vi "Dashboard Main.vi"() -> ()   [LabVIEW 2014]
uses:
  <vilib>/event_ctls.llb/eventvkey.ctl
  <vilib>/Utility/config.llb/NI_LVConfig.lvlib
  <vilib>/Utility/config.llb/Write Key (I32).vi
  <vilib>/Rock Robotics/WPI/Dashboard/WPI_DashboardLogging Global.vi
  <vilib>/Utility/config.llb/Write Key (String).vi
panel:
  in  "TCP":refnum<k5>
  out "Camera IP":string
  out "Image Message":string="Timeout in Camera Communications"
  in  "Dashboard Tab":T1(tab)
  out "RightPwr":dbl(slide) scale=-100.0..100.0
  out "RightSpd":dbl(slide) scale=-12.0..12.0
  out "LeftSpd":dbl(slide) scale=-12.0..12.0
  out "LeftPwr":dbl(slide) scale=-100.0..100.0
  in  "Camera Settings":T2={"Frame Rate"=30, "Compression"=30, "Size"=1} {"Frame Rate" scale=1.0..30.0; "Size" items=["640x480", "320x240", "160x120"]}
  out "MotorChart R":cluster{"Numeric":dbl, "Numeric":dbl}(graph)
  out "MotorChart L":T3(graph)
  out "MotorSliders R":cluster{"MotorSlide1":dbl, "MotorSlide2":dbl} {"MotorSlide2" scale=-1.0..1.0 scale format="%#_2e"; "MotorSlide1" scale=-1.0..1.0 scale format="%#_2e"}
  out "MotorSliders L":T4 {"MotorSlide4 2" scale=0.0..14.0 scale format="%#_2e"; "MotorSlide2" scale=-1.0..1.0 scale format="%#_2e"; "MotorSlide1" scale=-1.0..1.0 scale format="%#_2e"}
  out "JS1 Z":dbl(slide) scale=-1.0..1.0 scale format="%#_2e"
  out "JS1 Graph":cluster{"X":dbl, "Y":dbl}[](graph)
  out "JS1 Buttons":T5
  out "JS2 Z":dbl(slide) scale=-1.0..1.0 scale format="%#_2e"
  out "JS2 Graph":cluster{"X":dbl, "Y":dbl}[](graph)
  out "JS2 Buttons":T5
  out "Mode":T6(ring)=enum."Auto Disabled"
  in  "DB Camera Config":bool
  out "fps":dbl format="%#.1g"
  out "Mbps":dbl format="%#.1g"
  out "Mbps 2":bool
  in  "DB/String 9":string
  in  "DB/String 8":string
  in  "DB/String 7":string
  in  "DB/String 6":string
  in  "DB/String 5":string
  in  "DB/String 4":string
  in  "DB/String 3":string
  in  "DB/String 2":string
  in  "DB/String 1":string
  in  "DB/String 0":string
  in  "DB/Slider 0":dbl(slide) scale=0.0..5.0
  in  "DB/Slider 1":dbl(slide) scale=0.0..5.0
  in  "DB/Slider 2":dbl(slide) scale=0.0..5.0
  in  "DB/Slider 3":dbl(slide) scale=0.0..5.0
  out "DB/LED 3":bool
  out "DB/LED 2":bool
  out "DB/LED 1":bool
  out "DB/LED 0":bool
  in  "DB/Button 3":bool
  in  "DB/Button 2":bool
  in  "DB/Button 1":bool
  in  "DB/Button 0":bool caption="New Name"
  in  "Test Slider":dbl(slide) scale=0.0..100.0 scale format="%#_3g"
  in  "On/Off":bool caption="Solenoid"
  in  "Test Name":u16(ring) items=["Select the test to run...", "Example Test", "-------------------------------", "List of tests is built in robot code.", "Replace with your own automated tests."]
  in  "Test Tree":string(tree)
  in  "Motor":cluster{"Value":dbl, "Enable":bool} {"Value" scale=-1.0..1.0 scale format="%#_3g"}
  out "Progress":T7 {"Test Progress" scale=0.0..100.0}
  in  "Rev/Fwd":cluster{"Forward":bool, "Reverse":bool}
  in  "Test Ring":u16(ring) items=["Monochrome", "Color"]
  in  "Listbox":i32(listbox)
  out "Tree":string(tree)
  out "Boolean":bool
  # "Left"
  # "Front"
  # "Right"
  # "Battery"
  # "This tab is a great place for autonomous settings and robot-specific values.\nPlace controls and indicators inside this tab and match name to\nDashboard Variables on robot. You can also delete this comment."
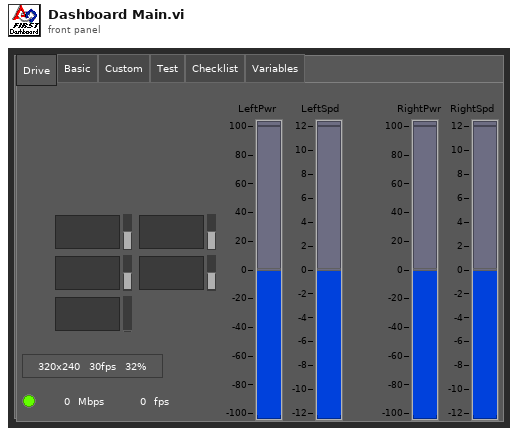
[diagram p1: front panel]
types:
  T1 = enum32{"Drive", "Basic", "Custom", "Test", "Checklist", "Variables"}
  T2 = cluster{"Frame Rate":i32, "Compression":i32, "Size":u16}
  T3 = cluster{"Numeric":dbl, "Numeric":dbl, "Battery V":dbl}
  T4 = cluster{"MotorSlide1":dbl, "MotorSlide2":dbl, "MotorSlide4 2":dbl}
  T5 = cluster{bool, bool, bool, bool, bool, bool, bool, bool, bool, bool, bool, bool}
  T6 = enum8{"Tele-Op Disabled", "Tele-Op Enabled", "Auto Disabled", "Auto Enabled", "Test Disabled", "Test Enabled", "Disconnected", "No Code", "E-Stop"}
  T7 = cluster{"Test Progress":u8, "Test Progress Text":string}
  T8 = typedef "Image Type" = u32
  T9 = typedef "IMAQ Image.ctl" = refnum<image>
  T10 = cluster{"Error Strings":string, "Disable Counts":cluster{u16, u16}, "Rail Faults":cluster{u16, u16, u16}, "Robot IP":string, "DB Mode":u8, "Event Info":cluster{"Name":string, "Type":u8, "Number":u16, "Replay":u8}, "Camera Addr":string}
  T11 = cluster{"Storage":cluster{"Disk Free":u64, "RAM Block":u32, "RAM free":u32}, "CPU Utilization":cluster{"CPU % ISR":sgl, "CPU % Time Crit":sgl, "CPU % Timed Str":sgl, "CPU % High":sgl, "CPU % Above":sgl, "CPU % Normal":sgl, "CPU % Low":sgl}, "CAN":cluster{"% Bus Utilization":sgl, "Bus Off Cnt":u32, "TX_FIFO Full Cnt":u32, "Receive Error Cnt":u8, "Transmit Error Cnt":u8}, "HID":cluster{"HID Outputs":u32, "Rumble Low":u16, "Rumble High":u16}[]}
  T12 = cluster{"Status bits":cluster{"Test Mode":bool, "Autonomous":bool, "Enabled":bool, "Code Start":bool, "Brownout":bool, "Reserved 2":bool, "Reserved 3":bool, "E-Stop":bool}, "Code Trace":cluster{"Disabled":bool, "TeleOp":bool, "Auto":bool, "Test":bool}, "Controller Type":enum16{"unknown", "cRIO", "roboRio"}, "Code?":enum16{"unknown", "noCode", "code"}, "Battery V":dbl}
  T13 = cluster{"Control Bits":cluster{"TestMode":bool, "Autonomous":bool, "Enabled":bool, "FMS Present":bool, bool, bool, bool, "E-Stop":bool}, "Team Station ":u8, "Countdown":sgl, "Joystick Values":cluster{"Axes":dbl[], "Buttons":bool[], "POVs":i16[]}[]}
  T14 = cluster{"Axes":dbl[], "Buttons":bool[], "POVs":i16[]}[]
  T15 = cluster{"Axes":dbl[], "Buttons":bool[], "POVs":i16[]}
  T16 = cluster{"Buttons[0]":bool, "Buttons[1]":bool, "Buttons[2]":bool, "Buttons[3]":bool, "Buttons[4]":bool, "Buttons[5]":bool, "Buttons[6]":bool, "Buttons[7]":bool, "Buttons[8]":bool, "Buttons[9]":bool, "Buttons[10]":bool, "Buttons[11]":bool}
  T17 = typedef "NI_LVConfig.lvlib/Config Data RefNum.ctl" = refnum<k1>
  T18 = cluster{"Operation":enum16{"Update", "Clear"}, "Color Box":u32}[]
  T19 = typedef "eventvkey.ctl" = enum16{"ASCII", "Enter", "Return", "Shift", "Ctrl", "Alt", "Cmd", "Opt", "Caps", "NumLock", "Clear", "Break", "Up", "Down", "Left", "Right", "Insert", "Delete", "Home", "End", "PageUp", "PageDown", "Escape", "Help", "Pause", "ScrollLock", "F1", "F2", "F3", "F4", "F5", "F6", "F7", "F8", "F9", "F10", "F11", "F12", "F13", "F14", "F15", "F16", "F17", "F18", "F19", "F20", "F21", "F22", "F23", "F24", "Play", "VolumeUp", "VolumeDown", "Mute", "Two Byte Char"}
  T20 = cluster{"Image Size":bool, "Image Type":bool, "Pixel Value":bool, "ROI Information":bool, "Zoom Factor":bool}
  T21 = enum8{"Enabled", "Disabled", "Disabled and Grayed Out"}
  T22 = cluster{"Operation":enum16{"Update", "Clear"}, "Color Box":u32}
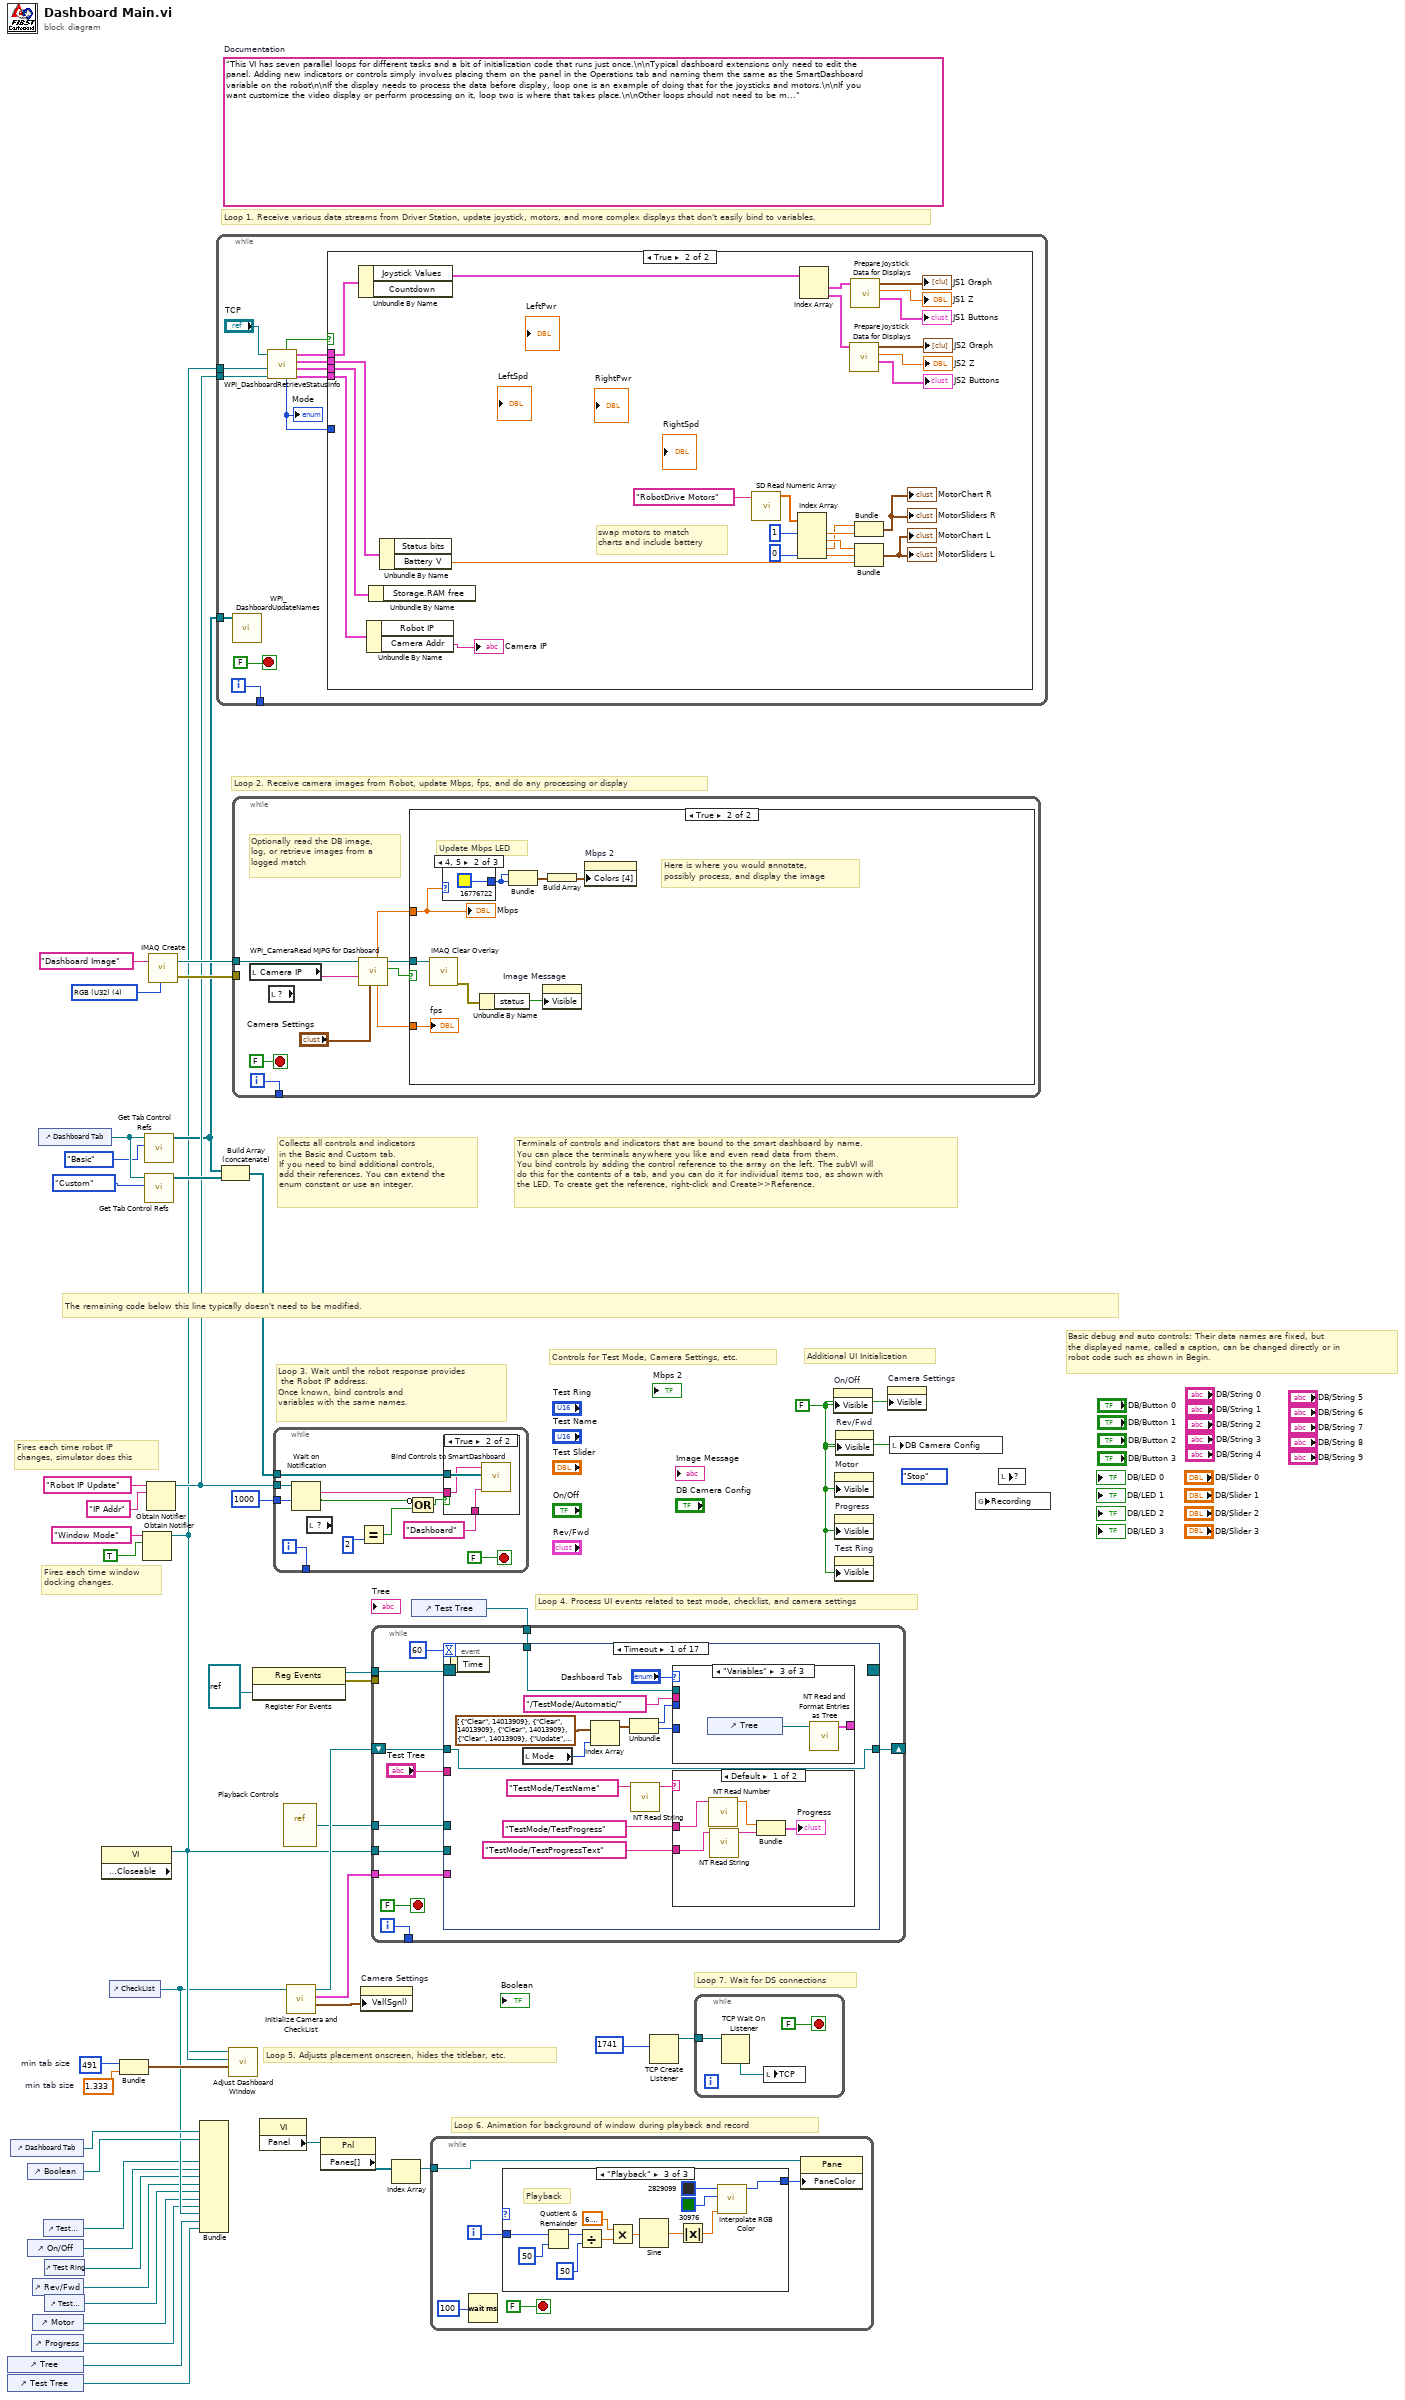
[diagram p0: block diagram]
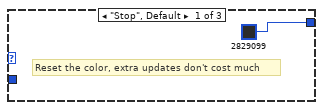
[diagram p3: hidden frame]
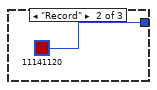
[diagram p4: hidden frame]
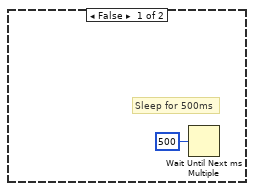
[diagram p6: hidden frame]
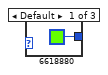
[diagram p7: hidden frame]
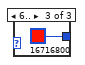
[diagram p8: hidden frame]
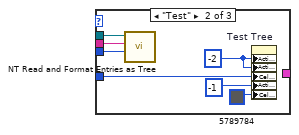
[diagram p10: hidden frame]
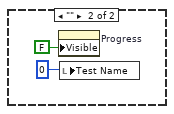
[diagram p11: hidden frame]
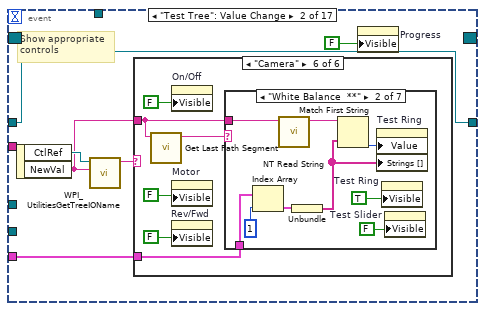
[diagram p12: hidden frame]
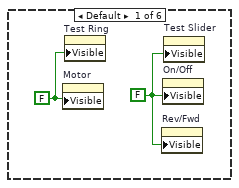
[diagram p13: hidden frame]
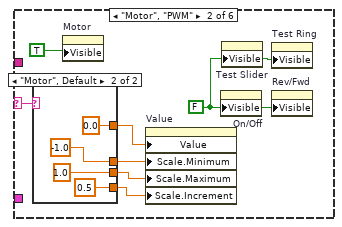
[diagram p14: hidden frame]
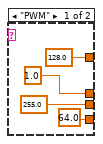
[diagram p15: hidden frame]
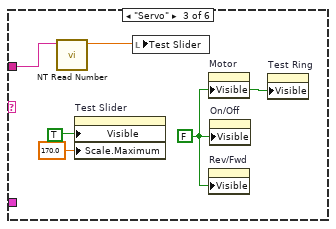
[diagram p16: hidden frame]
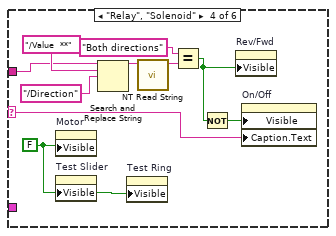
[diagram p17: hidden frame]
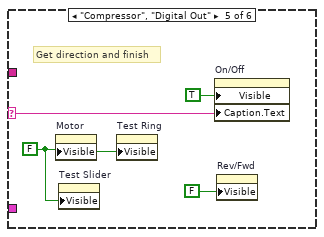
[diagram p18: hidden frame]
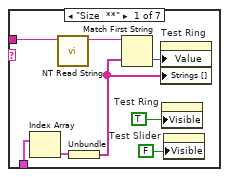
[diagram p19: hidden frame]
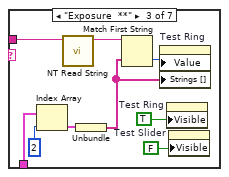
[diagram p20: hidden frame]
diagram:
  w22 = 491  # min tab size
  w21 = 1.333  # min tab size
  (unwired) enum32{"Stop", "Record", "Playback"}."Stop" ("Rec Mode")
  w6 = FALSE ("Visible")
  (unwired) "This VI has seven parallel loops for different tasks and a bit of initialization code that runs just once.\n\nTypical dashboard extensions only need to edit the panel. Adding new indicators or controls simply involves placing them on the panel in the Operations tab and naming them the same as the SmartDashboard variable on the robot\n\nIf the display needs to process the data before display, loop one is an example of doing that for the joysticks and motors.\n\nIf you want customize the video display or perform processing on it, loop two is where that takes place.\n\nOther loops should not need to be modified. They are pretty standard, and document the task they perform."  # Documentation
  w47 = T8 4 items=["Grayscale (U8)", "Grayscale (I16)", "Grayscale (SGL)", "Complex (CSG)", "RGB (U32)", "HSL (U32)", "RGB (U64)"] ("Image Type")
  # "Loop 7. Wait for DS connections"
  # "Basic debug and auto controls: Their data names are fixed, but\nthe displayed name, called a caption, can be changed directly or in\nrobot code such as shown in Begin."
  # "Controls for Test Mode, Camera Settings, etc."
  # "Additional UI Initialization"
  # "Loop 6. Animation for background of window during playback and record"
  # "Fires each time robot IP\nchanges, simulator does this"
  # "Fires each time window\ndocking changes."
  # "Collects all controls and indicators\nin the Basic and Custom tab.\nIf you need to bind additional controls,\nadd their references. You can extend the\nenum constant or use an integer."
  # "The remaining code below this line typically doesn't need to be modified."
  # "Loop 4. Process UI events related to test mode, checklist, and camera settings"
  # "Terminals of controls and indicators that are bound to the smart dashboard by name.\nYou can place the terminals anywhere you like and even read data from them.\nYou bind controls by adding the control reference to the array on the left. The subVI will\ndo this for the contents of a tab, and you can do it for individual items too, as shown with\nthe LED. To create get the reference, right-click and Create>>Reference."
  # "Loop 3. Wait until the robot response provides\n the Robot IP address.\nOnce known, bind controls and\nvariables with the same names."
  # "Loop 5. Adjusts placement onscreen, hides the titlebar, etc."
  # "Loop 1. Receive various data streams from Driver Station, update joystick, motors, and more complex displays that don't easily bind to variables."
  # "Loop 2. Receive camera images from Robot, update Mbps, fps, and do any processing or display"
  n1 = control-ref of="Tree"() -> (w15:refnum<vi>)
  n2 = control-ref of="Test Tree"() -> (w14:refnum<vi>)
  n3 = control-ref of="Dashboard Tab"() -> (w23:refnum<vi>)
  n4 = control-ref of="Boolean"() -> (w19:refnum<vi>)
  n5 = control-ref of="On/Off"() -> (w10:refnum<vi>)
  n6 = control-ref of="Progress"() -> (w7:refnum<vi>)
  n7 = control-ref of="Rev/Fwd"() -> (w8:refnum<vi>)
  n8 = control-ref of="Motor"() -> (w12:refnum<vi>)
  n9 = control-ref of="Dashboard Tab"() -> (w26:refnum<vi>)
  n10 = control-ref of="Test Slider"() -> (w11:refnum<vi>)
  n11 = control-ref of="Test Ring"() -> (w9:refnum<vi>)
  n12 = control-ref of="Test Name"() -> (w13:refnum<vi>)
  n13 = property class="VI" props=["Front Panel.Closeable"]() -> (reference out=w27:refnum<vi>)  [unwired: 2 in, 2 out]
  n14 = control-ref of="CheckList"() -> (w16:refnum<vi>)
  n15 = Bundle("min tab size"=w22, "min tab size"=w21) -> (w20:cluster{"min tab size":i32, "min tab size":dbl})  [unwired: 1 in]
  n16 = Obtain Notifier(name (unnamed)="Window Mode", notification data type=TRUE) -> (notifier out=w3:refnum<notifier>)  [unwired: 2 in, 2 out]
  n17 = call <vilib>:"Get Tab Control Refs.vi"("Page Index"=T1."Basic" ("Dashboard Tab"), "TabControl in"=w26) -> ("ControlsOnPage"=w4:refnum<vi>[])  [unwired: 9 in]
  n18 = call <vilib>:"Get Tab Control Refs.vi"("Page Index"=T1."Custom" ("Dashboard Tab"), "TabControl in"=w26) -> ("ControlsOnPage"=w25:refnum<vi>[])  [unwired: 9 in]
  n19 = Obtain Notifier(name (unnamed)="Robot IP Update", notification data type="IP Addr" ("name (unnamed)")) -> (notifier out=w5:refnum<notifier>)  [unwired: 2 in, 2 out]
  n20 = call "IMAQ Create"("Image Name"="Dashboard Image", "Image Type"=w47) -> ("New Image"=w45:T9, "error out"=w44:errorcluster)  [unwired: 2 in, 1 out]
  n21 = Bundle("Dashboard Tab"=w23, "Boolean"=w19, "Test Slider"=w11, "On/Off"=w10, "Test Ring"=w9, "Rev/Fwd"=w8, "Test Name"=w13, "Motor"=w12, "Progress"=w7, "CheckList"=w16, "Tree"=w15, "Test Tree"=w14) -> ()  [unwired: 4 in, 1 out]
  n22 = while {
    tunnel: [w58] -> _
    tunnel: w5 -> [w52]
    tunnel: w4 -> [w51]
    tunnel: w3 -> [w48]
    i -> [w58]
    stop <- FALSE stop-if-true
    n23 = call <vilib>:"WPI_DashboardUpdateNames.vi"("Controls on Tab"=w51) -> ()  [unwired: 11 in]
    n24 = call <vilib>:"WPI_DashboardRetrieveStatusInfo.vi"("Binding Refnum"=w52, "Window Mode Notifier"=w48, "TCP Cnx"="TCP") -> ("Power and Errors"=w53:T10, "Robot Metrics"=w56:T11, "Status Info"=w57:T12, "Control Info"=w54:T13, "Robot Mode"=w50:T6, "Process?"=w55:bool)  [unwired: 3 in]
    "Mode" <- w50
    n25 = case shown="True" w55 {
      tunnel: w57 -> [_ w84]
      tunnel: w56 -> [_ w83]
      tunnel: w54 -> [_ w82]
      tunnel: w53 -> [_ w81]
      tunnel: w50 -> [_ _]
      frame False {
      }
      frame True {
        # "swap motors to match\ncharts and include battery"
        n26 = Unbundle By Name(w82) -> ("Joystick Values"=w69:T14)  [unwired: 1 out]
        n27 = Unbundle By Name(w81) -> ("Camera Addr"=→"Camera IP":string)  [unwired: 1 out]
        n28 = Unbundle By Name(w83) -> ()  [unwired: 1 out]
        n29 = Unbundle By Name(w84) -> ("Battery V"=w70:dbl)  [unwired: 1 out]
        n30 = call <vilib>:"SD Read Numeric Array.vi"("Name"="RobotDrive Motors") -> ("Numeric Array"=w72:dbl[])  [unwired: 8 in, 2 out]
        n31 = Index Array(array=w72, index #1=1, index #4=0) -> (element #1=w76:dbl, element #2=w77:dbl, element #3=w75:dbl, element #4=w80:dbl)  [unwired: 2 in]
        n32 = Index Array(array=w69) -> (element #1=w68:T15, element #2=w63:T15)  [unwired: 2 in]
        n33 = call "Prepare Joystick Data for Displays.vi"("Joystick Values"=w63) -> ("Buttons"=→"JS2 Buttons":T16, "Z Axis"=→"JS2 Z":dbl, "Cartesian Data"=→"JS2 Graph":cluster{"X axis":dbl, "X axis":dbl}[])  [unwired: 8 in]
        n34 = call "Prepare Joystick Data for Displays.vi"("Joystick Values"=w68) -> ("Buttons"=→"JS1 Buttons":T16, "Z Axis"=→"JS1 Z":dbl, "Cartesian Data"=→"JS1 Graph":cluster{"X axis":dbl, "X axis":dbl}[])  [unwired: 8 in]
        n35 = Bundle("Numeric"=w75, "Numeric"=w76) -> (→"MotorChart R" →"MotorSliders R":cluster{"Numeric":dbl, "Numeric":dbl})  [unwired: 1 in]
        n36 = Bundle("Numeric"=w77, "Numeric"=w80, "Battery V"=w70) -> (→"MotorChart L" →"MotorSliders L":T3)  [unwired: 1 in]
      }
    }
  }
  n37 = Build Array (concatenate)(w4, w25) -> (w24:refnum<vi>[])
  n38 = call "Adjust Dashboard Window.vi"("Size Constraints"=w20, "VI"=w27, "Notifier in"=w3) -> ()  [unwired: 9 in]
  n39 = while {
    tunnel: w45 -> [w91]
    tunnel: w44 -> [_]
    tunnel: [w92] -> _
    i -> [w92]
    stop <- FALSE stop-if-true
    # "Optionally read the DB image,\nlog, or retrieve images from a\nlogged match"
    n40 = local read "Camera IP"() -> (w85:string)
    n41 = local read item#-1() -> ()  [unwired: 1 out]
    n42 = call <vilib>:"WPI_CameraRead MJPG for Dashboard.vi"("Camera Settings"="Camera Settings", "Camera IP"=w85, "Refnum in"=w91) -> ("Active"=w89:bool, "Refnum out"=w90:T9, "FPS"=w88:dbl, "Bandwidth (Mbps)"=w87:dbl)  [unwired: 5 in]
    n43 = case shown="True" w89 {
      tunnel: w90 -> [_ w97]
      tunnel: w87 -> [_ w96]
      tunnel: w88 -> [_ w95]
      frame False {
        # "Sleep for 500ms"
        n44 = Wait Until Next ms Multiple(millisecond multiple=u32 500) -> ()  [unwired: 1 out]
      }
      frame True {
        # "Here is where you would annotate,\npossibly process, and display the image"
        # "Update Mbps LED"
        n45 = call "IMAQ Clear Overlay"("Image"=w97) -> ("error out"=w101:errorcluster)  [unwired: 2 in, 8 out]
        n46 = case shown="4, 5" w96 {
          tunnel: [u32 6618880 ("Color Box") u32 16776722 ("Color Box") u32 16716800 ("Color Box")] -> w98
          frame Default {
          }
          frame 4, 5 {
          }
          frame 6.. {
          }
        }
        n47 = Unbundle By Name(w101) -> ("status"=w102:bool)
        n48 = Bundle("Color Box"=w98, "Color Box"=w98) -> (w100:cluster{"Color Box":u32, "Color Box":u32})  [unwired: 1 out]
        n49 = property on="Image Message" class="Str"("Visible"=w102) -> ()  [unwired: 2 in, 2 out]
        n50 = Build Array(w100) -> (w99:cluster{"Color Box":u32, "Color Box":u32}[])
        n51 = property on="Mbps 2" class="Bool (strict)"("Colors [4]"=w99) -> ()  [unwired: 2 in, 2 out]
        "Mbps" <- w96
        "fps" <- w95
      }
    }
  }
  n52 = register-events(refnum<vi> refnum) -> (reference out=w31:refnum<event-registration>, error out=w30:errorcluster)  [unwired: 2 in]
  n53 = property class="VI"() -> ("Panel"=w34:refnum<vi>)  [unwired: 2 in, 2 out]
  n54 = while {
    tunnel: w24 -> [w116]
    tunnel: w5 -> [w114]
    tunnel: [w112] -> _
    tunnel: u32 1000 ("milliseconds to wait") -> [w111]
    i -> [w112]
    stop <- FALSE stop-if-true
    n55 = Wait on Notification(notifier=w114, timeout in ms (-1)=w111) -> (notification=w113:string, timed out?=w109:bool)  [unwired: 2 in, 2 out]
    n56 = local read item#-1() -> ()  [unwired: 1 out]
    n57 = Equal?(y=u16 2 ("Rec Mode")) -> (x = y?=w108:bool)  [unwired: 1 in]
    n58 = Compound Arithmetic op=OR(invert w109, w108) -> (w110:bool)
    n59 = case shown="True" w110 {
      tunnel: w116 -> [_ w119]
      tunnel: w113 -> [_ w118]
      tunnel: "Dashboard" -> [_ w117]
      frame False {
      }
      frame True {
        n60 = call <vilib>:"Bind Controls to SmartDashboard.vi"("Client Name"=w117, "Bound Control Refs"=w119, "Server IP Address"=w118) -> ()  [unwired: 9 in]
      }
    }
  }
  n61 = vi-ref "Playback Controls.vi"() -> (w32:refnum<vi>)
  n62 = call "Initialize Camera and CheckList.vi"("ListBox in"=w16) -> ("Cluster"=w38:cluster{"value":i32, "value":i32, "index":i32}, "Array"=w39:cluster{string[]}[], "File Refnum"=w37:T17)  [unwired: 8 in]
  n63 = property class="Pnl"(reference=w34) -> ("Panes[]"=w35:refnum<vi>[])  [unwired: 1 in, 2 out]
  n64 = property on="Camera Settings" class="Clust (strict)"("Val(Sgnl)"=w38) -> ()  [unwired: 2 in, 2 out]
  n65 = Index Array(array=w35) -> (element=w33:refnum<vi>)  [unwired: 1 in]
  n66 = control-ref of="Test Tree"() -> (w36:refnum<vi>)
  n67 = while {
    tunnel: w39 -> [w127]
    shift-right: [w126] -> _
    shift-left: w37 -> [w125]
    tunnel: [w124] -> _
    tunnel: w36 -> [w123]
    tunnel: w32 -> [w122]
    tunnel: w31 -> [w121]
    tunnel: w30 -> [_]
    tunnel: w27 -> [w120]
    i -> [w124]
    stop <- FALSE stop-if-true
    n68 = event shown="[0] Timeout" {
      selector: w121 -> [_ _ _ _ _ _ _ _ _ _ _ _ _ _ _ _ _]
      dyn-events: [_ _ _ _ _ _ _ _ _ _ _ _ _ w363 _ _ _] -> _
      timeout: u32 60 ("milliseconds to wait") -> [_ _ _ _ _ _ _ _ _ _ _ _ _ _ _ _ _]
      tunnel: w123 -> [w139 _ _ _ _ _ _ _ _ _ _ _ _ _ _ _ _]
      tunnel: "Test Tree" -> [_ _ _ _ _ _ _ _ w334 w342 w344 w348 w356 _ _ _ _]
      tunnel: w127 -> [_ w161 _ _ _ _ w298 w328 _ _ _ _ _ _ _ _ _]
      tunnel: [w135 w160 w259 w264 w272 w284 w297 w321 w333 w340 w343 w347 w355 w365 w377 w378 w387] -> w126
      tunnel: w125 -> [w135 w160 w259 w264 w272 w284 w296 w321 w333 w340 w343 w347 w355 w365 w377 w378 w387]
      tunnel: w122 -> [_ _ _ _ _ _ _ _ _ _ _ _ _ w366 _ w381 _]
      tunnel: w120 -> [_ _ _ _ _ _ _ _ _ _ _ _ _ w361 _ _ _]
      event Timeout {
        n69 = event-data() -> ()  [unwired: 1 in, 1 out]
        n70 = local read "Mode"() -> (w138:T6)
        n71 = Index Array(array=T18 [{"Operation"=enum."Clear", "Color Box"=14013909}, {"Operation"=enum."Clear", "Color Box"=14013909}, {"Operation"=enum."Clear", "Color Box"=14013909}, {"Operation"=enum."Clear", "Color Box"=14013909}, {"Operation"=enum."Update", "Color Box"=14013909}, {"Operation"=enum."Update", "Color Box"=16777215}, {"Operation"=enum."Clear", "Color Box"=14013909}, {"Operation"=enum."Clear", "Color Box"=14013909}, {"Operation"=enum."Clear", "Color Box"=14013909}], index=w138) -> (element=w133:T22)
        n72 = Unbundle(w133) -> ("Operation"=w132:enum16{"Update", "Clear"}, "Color Box"=w131:u32)
        n73 = call <vilib>:"NT Read String.vi"("Name"="TestMode/TestName") -> ("String"=w142:string)  [unwired: 9 in, 1 out]
        n74 = case shown="\"Variables\"" "Dashboard Tab" {
          tunnel: w139 -> [_ w150 _]
          tunnel: "/TestMode/Automatic/" ("Name Pattern") -> [_ w149 _]
          tunnel: w132 -> [_ w148 _]
          tunnel: [_ _ w152] -> _
          tunnel: w131 -> [_ w144 _]
          frame "Custom", Default {
          }
          frame "Test" {
            w147 = -2 ("Active Item:Row Number")
            n75 = call <vilib>:"NT Read and Format Entries as Tree.vi"("Operation"=w148, "Name Pattern"=w149, "Tree Refnum"=w150) -> ()  [unwired: 7 in, 2 out]
            n76 = property on="Test Tree" class="Tree (strict)"("Active Item Row Number"=w147, "ActiveColNum"=w147, "CellBG"=w144, "Active Item Row Number"=-1 ("Active Item:Row Number"), "CellBG"=u32 5789784 ("Color Box")) -> ()  [unwired: 2 in, 2 out]
          }
          frame "Variables" {
            n77 = control-ref of="Tree"() -> (w151:refnum<vi>)
            n78 = call <vilib>:"NT Read and Format Entries as Tree.vi"("Tree Refnum"=w151) -> ("Formatted Strings"=w152:cluster{"Name":string, "Value":string}[])  [unwired: 9 in, 1 out]
          }
        }
        n79 = case shown="Default" w142 {
          tunnel: "TestMode/TestProgress" ("Name") -> [w154 _]
          tunnel: "TestMode/TestProgressText" ("Name") -> [w153 _]
          frame Default {
            n80 = call <vilib>:"NT Read Number.vi"("Name"=w154) -> ("Numeric"=w155:dbl)  [unwired: 9 in, 1 out]
            n81 = call <vilib>:"NT Read String.vi"("Name"=w153) -> ("String"=w156:string)  [unwired: 9 in, 1 out]
            n82 = Bundle("Numeric"=w155, "String"=w156) -> (→"Progress":cluster{"Numeric":dbl, "String":string})  [unwired: 1 in]
          }
          frame "" {
            n83 = property on="Progress" class="Clust (strict)"("Visible"=FALSE) -> ()  [unwired: 2 in, 2 out]
            n84 = local write "Test Name"(u16 0) -> ()
          }
        }
      }
      event "Test Tree": Value Change {
        # "Show appropriate\ncontrols"
        n85 = event-data() -> ("CtlRef"=w164:refnum<vi>, "NewVal"=w162:string)  [unwired: 1 in]
        n86 = call <vilib>:"WPI_UtilitiesGetTreeIOName.vi"("NewVal"=w162, "TreeControl in"=w164) -> ("I/O Name"=w165:string)  [unwired: 9 in]
        n87 = case shown="\"Camera\"" w165 {
          selector: w165 -> [_ w172 _ w190 w199 _]
          tunnel: w162 -> [_ _ w187 w189 _ w206]
          tunnel: w161 -> [_ _ _ _ _ w205]
          frame Default {
            w167 = FALSE ("Visible")
            w166 = FALSE ("Visible")
            n88 = property on="Motor" class="Clust (strict)"("Visible"=w166) -> ()  [unwired: 2 in, 2 out]
            n89 = property on="Test Ring" class="Ring (strict)"("Visible"=w166) -> ()  [unwired: 2 in, 2 out]
            n90 = property on="Rev/Fwd" class="Clust (strict)"("Visible"=w167) -> ()  [unwired: 2 in, 2 out]
            n91 = property on="On/Off" class="Bool (strict)"("Visible"=w167) -> ()  [unwired: 2 in, 2 out]
            n92 = property on="Test Slider" class="Slide (strict)"("Visible"=w167) -> ()  [unwired: 2 in, 2 out]
          }
          frame "Motor", "PWM" {
            w173 = FALSE ("Visible")
            n93 = case shown="\"Motor\", Default" w172 {
              tunnel: [1.0 ("Value") -1.0 ("Value")] -> w171
              tunnel: [255.0 ("Value") 1.0 ("Value")] -> w170
              tunnel: [128.0 ("Value") 0.0 ("Value")] -> w169
              tunnel: [64.0 ("Value") 0.5 ("Value")] -> w168
              frame "PWM" {
              }
              frame "Motor", Default {
              }
            }
            n94 = property on="Motor" class="Clust (strict)"("Visible"=TRUE) -> ()  [unwired: 2 in, 2 out]
            n95 = property on="Value" class="Slide (strict)"("Value"=w169, "Scale.Minimum"=w171, "Scale.Maximum"=w170, "Scale.Increment"=w168) -> ()  [unwired: 2 in, 2 out]
            n96 = property on="On/Off" class="Bool (strict)"("Visible"=w173) -> ()  [unwired: 2 in, 2 out]
            n97 = property on="Test Slider" class="Slide (strict)"("Visible"=w173) -> ()  [unwired: 2 in, 2 out]
            n98 = property on="Test Ring" class="Ring (strict)"("Visible"=w173) -> ()  [unwired: 2 in, 2 out]
            n99 = property on="Rev/Fwd" class="Clust (strict)"("Visible"=w173) -> ()  [unwired: 2 in, 2 out]
          }
          frame "Servo" {
            w185 = FALSE ("Visible")
            n100 = call <vilib>:"NT Read Number.vi"("Name"=w187) -> ("Numeric"=w186:dbl)  [unwired: 9 in, 1 out]
            n101 = property on="Test Slider" class="Slide (strict)"("Visible"=TRUE, "Scale.Maximum"=170.0 ("Scale.Range:Maximum")) -> ()  [unwired: 2 in, 2 out]
            n102 = local write "Test Slider"(w186) -> ()
            n103 = property on="Motor" class="Clust (strict)"("Visible"=w185) -> ()  [unwired: 2 in, 2 out]
            n104 = property on="Rev/Fwd" class="Clust (strict)"("Visible"=w185) -> ()  [unwired: 2 in, 2 out]
            n105 = property on="On/Off" class="Bool (strict)"("Visible"=w185) -> ()  [unwired: 2 in, 2 out]
            n106 = property on="Test Ring" class="Ring (strict)"("Visible"=w185) -> ()  [unwired: 2 in, 2 out]
          }
          frame "Relay", "Solenoid" {
            w188 = FALSE ("Visible")
            n107 = property on="Motor" class="Clust (strict)"("Visible"=w188) -> ()  [unwired: 2 in, 2 out]
            n108 = property on="Test Slider" class="Slide (strict)"("Visible"=w188) -> ()  [unwired: 2 in, 2 out]
            n109 = Search and Replace String(input string=w189, search string="/Value  **", replace string="/Direction") -> (result string=w195:string)  [unwired: 5 in, 3 out]
            n110 = property on="Test Ring" class="Ring (strict)"("Visible"=w188) -> ()  [unwired: 2 in, 2 out]
            n111 = call <vilib>:"NT Read String.vi"("Name"=w195) -> ("String"=w193:string)  [unwired: 9 in, 1 out]
            n112 = Equal?(x="Both directions", y=w193) -> (x = y?=w191:bool)
            n113 = Not(x=w191) -> (.not. x?=w192:bool)
            n114 = property on="Rev/Fwd" class="Clust (strict)"("Visible"=w191) -> ()  [unwired: 2 in, 2 out]
            n115 = property on="On/Off" class="Bool (strict)"("Visible"=w192, "Caption.Text"=w190) -> ()  [unwired: 2 in, 2 out]
          }
          frame "Compressor", "Digital Out" {
            w198 = FALSE ("Visible")
            # "Get direction and finish"
            n116 = property on="Motor" class="Clust (strict)"("Visible"=w198) -> ()  [unwired: 2 in, 2 out]
            n117 = property on="Test Slider" class="Slide (strict)"("Visible"=w198) -> ()  [unwired: 2 in, 2 out]
            n118 = property on="Test Ring" class="Ring (strict)"("Visible"=w198) -> ()  [unwired: 2 in, 2 out]
            n119 = property on="On/Off" class="Bool (strict)"("Visible"=TRUE, "Caption.Text"=w199) -> ()  [unwired: 2 in, 2 out]
            n120 = property on="Rev/Fwd" class="Clust (strict)"("Visible"=FALSE) -> ()  [unwired: 2 in, 2 out]
          }
          frame "Camera" {
            n121 = call <vilib>:"Get Last Path Segment.vi"("String in"=w206) -> ("String out"=w207:string)  [unwired: 10 in]
            n122 = property on="On/Off" class="Bool (strict)"("Visible"=FALSE) -> ()  [unwired: 2 in, 2 out]
            n123 = property on="Motor" class="Clust (strict)"("Visible"=FALSE) -> ()  [unwired: 2 in, 2 out]
            n124 = property on="Rev/Fwd" class="Clust (strict)"("Visible"=FALSE) -> ()  [unwired: 2 in, 2 out]
            n125 = case shown="\"White Balance  **\"" w207 {
              tunnel: w206 -> [w213 w222 w231 w240 w249 _ w255]
              tunnel: w205 -> [w211 w219 w228 w237 w246 _ _]
              frame "Size  **" {
                n126 = Index Array(array=w211) -> (element=w210:cluster{string[]})  [unwired: 1 in]
                n127 = call <vilib>:"NT Read String.vi"("Name"=w213) -> ("String"=w212:string)  [unwired: 9 in, 1 out]
                n128 = Unbundle(w210) -> (w208:string[])
                n129 = Match First String(2:w208, 3:w212) -> (0:w209:i32)  [unwired: 1 out]
                n130 = property on="Test Ring" class="Ring (strict)"("Value"=w209, "Strings []"=w208) -> ()  [unwired: 2 in, 2 out]
                n131 = property on="Test Ring" class="Ring (strict)"("Visible"=TRUE) -> ()  [unwired: 2 in, 2 out]
                n132 = property on="Test Slider" class="Slide (strict)"("Visible"=FALSE) -> ()  [unwired: 2 in, 2 out]
              }
              frame "White Balance  **" {
                n133 = Index Array(array=w219, index=1) -> (element=w220:cluster{string[]})
                n134 = call <vilib>:"NT Read String.vi"("Name"=w222) -> ("String"=w221:string)  [unwired: 9 in, 1 out]
                n135 = Unbundle(w220) -> (w217:string[])
                n136 = Match First String(2:w217, 3:w221) -> (0:w216:i32)  [unwired: 1 out]
                n137 = property on="Test Ring" class="Ring (strict)"("Value"=w216, "Strings []"=w217) -> ()  [unwired: 2 in, 2 out]
                n138 = property on="Test Ring" class="Ring (strict)"("Visible"=TRUE) -> ()  [unwired: 2 in, 2 out]
                n139 = property on="Test Slider" class="Slide (strict)"("Visible"=FALSE) -> ()  [unwired: 2 in, 2 out]
              }
              frame "Exposure  **" {
                n140 = Index Array(array=w228, index=2) -> (element=w229:cluster{string[]})
                n141 = call <vilib>:"NT Read String.vi"("Name"=w231) -> ("String"=w230:string)  [unwired: 9 in, 1 out]
                n142 = Unbundle(w229) -> (w225:string[])
                n143 = Match First String(2:w225, 3:w230) -> (0:w226:i32)  [unwired: 1 out]
                n144 = property on="Test Ring" class="Ring (strict)"("Value"=w226, "Strings []"=w225) -> ()  [unwired: 2 in, 2 out]
                n145 = property on="Test Ring" class="Ring (strict)"("Visible"=TRUE) -> ()  [unwired: 2 in, 2 out]
                n146 = property on="Test Slider" class="Slide (strict)"("Visible"=FALSE) -> ()  [unwired: 2 in, 2 out]
              }
              frame "Exposure Priority  **" {
                n147 = Index Array(array=w237, index=3) -> (element=w238:cluster{string[]})
                n148 = call <vilib>:"NT Read String.vi"("Name"=w240) -> ("String"=w239:string)  [unwired: 9 in, 1 out]
                n149 = Unbundle(w238) -> (w234:string[])
                n150 = Match First String(2:w234, 3:w239) -> (0:w235:i32)  [unwired: 1 out]
                n151 = property on="Test Ring" class="Ring (strict)"("Value"=w235, "Strings []"=w234) -> ()  [unwired: 2 in, 2 out]
                n152 = property on="Test Ring" class="Ring (strict)"("Visible"=TRUE) -> ()  [unwired: 2 in, 2 out]
                n153 = property on="Test Slider" class="Slide (strict)"("Visible"=FALSE) -> ()  [unwired: 2 in, 2 out]
              }
              frame "Color Enable  **" {
                n154 = Index Array(array=w246, index=4) -> (element=w247:cluster{string[]})
                n155 = call <vilib>:"NT Read String.vi"("Name"=w249) -> ("String"=w248:string)  [unwired: 9 in, 1 out]
                n156 = Unbundle(w247) -> (w243:string[])
                n157 = Match First String(2:w243, 3:w248) -> (0:w244:i32)  [unwired: 1 out]
                n158 = property on="Test Ring" class="Ring (strict)"("Value"=w244, "Strings []"=w243) -> ()  [unwired: 2 in, 2 out]
                n159 = property on="Test Ring" class="Ring (strict)"("Visible"=TRUE) -> ()  [unwired: 2 in, 2 out]
                n160 = property on="Test Slider" class="Slide (strict)"("Visible"=FALSE) -> ()  [unwired: 2 in, 2 out]
              }
              frame Default {
                n161 = property on="Test Ring" class="Ring (strict)"("Visible"=FALSE) -> ()  [unwired: 2 in, 2 out]
                n162 = property on="Test Slider" class="Slide (strict)"("Visible"=FALSE) -> ()  [unwired: 2 in, 2 out]
              }
              frame "Brightness  **", "Color Level  **", "Compression  **", "FPS  **", "Sharpness  **" {
                n163 = call <vilib>:"NT Read Number.vi"("Name"=w255) -> ("Numeric"=w254:dbl)  [unwired: 9 in, 1 out]
                n164 = local write "Test Slider"(w254) -> ()
                n165 = property on="Test Slider" class="Slide (strict)"("Visible"=TRUE, "Scale.Maximum"=100.0 ("Scale.Range:Maximum")) -> ()  [unwired: 2 in, 2 out]
                n166 = property on="Test Ring" class="Ring (strict)"("Visible"=FALSE) -> ()  [unwired: 2 in, 2 out]
              }
            }
          }
        }
        n167 = property on="Progress" class="Clust (strict)"("Visible"=FALSE) -> ()  [unwired: 2 in, 2 out]
      }
      event "Test Name": Mouse Enter {
        # "Populate the ring with the list of tests"
        n168 = event-data() -> ()  [unwired: 1 in, 1 out]
        n169 = call <vilib>:"NT Read String Array.vi"("Name"="TestMode/TestList") -> ("String Array"=w263:string[])  [unwired: 9 in, 1 out]
        n170 = Build Array (concatenate)("Select the test to run...", w263) -> (w262:string[])
        n171 = property on="Test Name" class="Ring (strict)"("Strings []"=w262) -> ()  [unwired: 2 in, 2 out]
      }
      event "Test Name": Value Change {
        w265 = FALSE ("Visible")
        # "Tell the robot the test name to run"
        n172 = event-data() -> ("NewVal"=w269:u16)  [unwired: 1 in]
        n173 = property on="Test Name" class="Ring (strict)"() -> ("Strings []"=w270:string[])  [unwired: 2 in, 2 out]
        n174 = local write "Progress"(T7 {"Test Progress"=0, "Test Progress Text"=""} ("Progress")) -> ()
        n175 = Index Array(array=w270, index=w269) -> (element=w268:string)
        n176 = call <vilib>:"NT Write String.vi"("String"=w268, "Name"="TestMode/TestName") -> ()  [unwired: 9 in, 1 out]
        n177 = property on="Progress" class="Clust (strict)"("Visible"=TRUE) -> ()  [unwired: 2 in, 2 out]
        n178 = property on="Motor" class="Clust (strict)"("Visible"=w265) -> ()  [unwired: 2 in, 2 out]
        n179 = property on="Test Slider" class="Slide (strict)"("Visible"=w265) -> ()  [unwired: 2 in, 2 out]
        n180 = property on="On/Off" class="Bool (strict)"("Visible"=w265) -> ()  [unwired: 2 in, 2 out]
        n181 = property on="Rev/Fwd" class="Clust (strict)"("Visible"=w265) -> ()  [unwired: 2 in, 2 out]
        n182 = property on="Test Ring" class="Ring (strict)"("Visible"=w265) -> ()  [unwired: 2 in, 2 out]
      }
      event "Listbox": Double Click {
        # "Shift clears all"
        # "Update symbols on the listbox"
        n183 = event-data() -> ("PlatMods.Shift"=w273:bool, "Row"=w275:i32)  [unwired: 1 in]
        n184 = case shown="True" w273 {
          tunnel: w275 -> [w279 _]
          tunnel: 1 -> [w278 _]
          frame False {
            n185 = property on="Listbox" class="LstBox (strict)"() -> ("Item Symbols"=w277:i32[])  [unwired: 2 in, 2 out]
            n186 = Replace Array Subset(array=w277, new element=w278, index=w279) -> (w276:i32[])
            n187 = property on="Listbox" class="LstBox (strict)"("Item Symbols"=w276) -> ()  [unwired: 2 in, 2 out]
          }
          frame True {
            w280 = 0 ("Top Row")
            n188 = property on="Listbox" class="LstBox (strict)"() -> ("Number of Rows"=w282:u32)  [unwired: 2 in, 2 out]
            n189 = Initialize Array(0, w282) -> (w281:i32[])
            n190 = property on="Listbox" class="LstBox (strict)"("Top Row"=w280, "Value"=w280, "Item Symbols"=w281) -> ()  [unwired: 2 in, 2 out]
          }
        }
      }
      event "Listbox": Key Down {
        # "Update symbols on the listbox\nLeft and right keys check and uncheck"
        n191 = event-data() -> ("VKey"=w286:T19)  [unwired: 1 in]
        n192 = case shown="\"Left\", \"Right\"" w286 {
          selector: w286 -> [w291 _]
          tunnel: eventvkey."Left" ("VKey") -> [w289 _]
          frame "Left", "Right" {
            n193 = Equal?(x=w289, y=w291) -> (x = y?=w290:bool)
            n194 = Select(t=0, s=w290, f=1) -> (s? t:f=w292:i32)
            n195 = property on="Listbox" class="LstBox (strict)"() -> ("Item Symbols"=w295:i32[])  [unwired: 2 in, 2 out]
            n196 = Replace Array Subset(array=w295, new element=w292, index="Listbox") -> (w294:i32[])
            n197 = property on="Listbox" class="LstBox (strict)"("Item Symbols"=w294) -> ()  [unwired: 2 in, 2 out]
          }
          frame Default {
          }
        }
      }
      event "DB Camera Config": Value Change {
        # "Show or hide the cluster of controls, store in ini file"
        n198 = event-data() -> ("NewVal"=w299:bool)  [unwired: 1 in]
        n199 = case shown="False" w299 {
          tunnel: w298 -> [w308 _]
          tunnel: [w301 w319] -> w297
          tunnel: w296 -> [w300 w319]
          frame False {
            w315 = "Camera"
            w318 = FALSE ("Visible")
            n200 = local read "Camera Settings"() -> (w307:T2)
            n201 = Index Array(array=w308) -> (element=w311:cluster{string[]})  [unwired: 1 in]
            n202 = Unbundle(w307) -> ("Frame Rate"=w306:i32, "Compression"=w305:i32, "Size"=w309:u16)
            n203 = Unbundle(w311) -> (w310:string[])
            n204 = Index Array(array=w310, index=w309) -> (element=w304:string)
            n205 = call-poly <vilib>:"Write Key.vi"("section"=w315, "value"=w304, "key"="Size", "refnum"=w300) -> ("refnum out"=w317:T17)  [unwired: 2 in, 5 out]
            n206 = call-poly <vilib>:"Write Key.vi"("section"=w315, "value"=w306, "key"="FrameRate", "refnum"=w317) -> ("refnum out"=w316:T17)  [unwired: 1 in, 6 out]
            n207 = property on="Camera Settings" class="Clust (strict)"("Visible"=w318) -> ()  [unwired: 2 in, 2 out]
            n208 = local write "DB Camera Config"(w318) -> ()
            n209 = call-poly <vilib>:"Write Key.vi"("section"=w315, "value"=w305, "key"="Compression", "refnum"=w316) -> ("refnum out"=w302:T17)  [unwired: 1 in, 6 out]
            n210 = call <vilib>:"Close Config Data.vi"("refnum"=w302) -> ("file path"=w303:path)  [unwired: 2 in, 8 out]
            n211 = call <vilib>:"Open Config Data.vi"("configuration file path"=w303) -> ("refnum"=w301:T17)  [unwired: 8 in, 2 out]
          }
          frame True {
            n212 = property on="Camera Settings" class="Clust (strict)"("Visible"=TRUE) -> ()  [unwired: 2 in, 2 out]
          }
        }
      }
      event "Camera Settings": Value Change {
        # "Update summary string when any elements of DB camera change"
        n213 = event-data() -> ("NewVal"=w332:T2)  [unwired: 1 in]
        n214 = Index Array(array=w328) -> (element=w327:cluster{string[]})  [unwired: 1 in]
        n215 = Unbundle(w332) -> ("Frame Rate"=w323:i32, "Compression"=w322:i32, "Size"=w325:u16)
        n216 = Unbundle(w327) -> (w326:string[])
        n217 = Index Array(array=w326, index=w325) -> (element=w324:string)
        n218 = Format Into String(format string="%s   %dfps   %d%%", w324, w323, w322) -> (resulting string=w329:string)  [unwired: 2 in, 1 out]
        n219 = Build Array(w329) -> (w330:string[])
        n220 = property on="DB Camera Config" class="Bool (strict)"("Strings [4]"=w330) -> ()  [unwired: 2 in, 2 out]
      }
      event "Motor.Enable": Value Change {
        # "When the test mode otor enable helper is set, update that\ntree row item's value"
        n221 = event-data() -> ("NewVal"=w338:bool)  [unwired: 1 in]
        n222 = Unbundle("Motor") -> ("Value"=w337:dbl)  [unwired: 1 out]
        n223 = Select(t=w337, s=w338, f=0.0) -> (s? t:f=w335:dbl)
        n224 = call <vilib>:"NT Write Number.vi"("Numeric"=w335, "Name"=w334) -> ()  [unwired: 9 in, 1 out]
      }
      event "Test Slider": Value Change {
        # "When the test mode slider helper is set, update that\ntree row item's value"
        n225 = event-data() -> ("NewVal"=w341:dbl)  [unwired: 1 in]
        n226 = call <vilib>:"NT Write Number.vi"("Numeric"=w341, "Name"=w342) -> ()  [unwired: 9 in, 1 out]
      }
      event "On/Off": Value Change {
        # "When the test mode on/off helper value is set, update that\ntree row item's value"
        n227 = event-data() -> ("NewVal"=w346:bool)  [unwired: 1 in]
        n228 = Boolean To (0,1)(Boolean=w346) -> (0, 1=w345:i16)
        n229 = call <vilib>:"NT Write Number.vi"("Numeric"=w345, "Name"=w344) -> ()  [unwired: 9 in, 1 out]
      }
      event "Rev/Fwd": Value Change {
        # "When the test mode helper value for relays is set, update that\ntree row item's value"
        n230 = event-data() -> ("NewVal.Forward"=w354:bool, "NewVal.Reverse"=w353:bool)  [unwired: 1 in]
        n231 = Boolean To (0,1)(Boolean=w354) -> (0, 1=w350:i16)
        n232 = Boolean To (0,1)(Boolean=w353) -> (0, 1=w352:i16)
        n233 = Negate(x=w352) -> (-x=w351:i16)
        n234 = Add(x=w350, y=w351) -> (x+y=w349:i16)
        n235 = call <vilib>:"NT Write Number.vi"("Numeric"=w349, "Name"=w348) -> ()  [unwired: 9 in, 1 out]
      }
      event "Test Ring": Value Change {
        # "When a test mode helper value is selected from the ring,\nset the tree item's variable to the string value"
        n236 = event-data() -> ("NewVal"=w358:u16)  [unwired: 1 in]
        n237 = property on="Test Ring" class="Ring (strict)"() -> ("Strings []"=w359:string[])  [unwired: 2 in, 2 out]
        n238 = Index Array(array=w359, index=w358) -> (element=w357:string)
        n239 = call <vilib>:"NT Write String.vi"("String"=w357, "Name"=w356) -> ()  [unwired: 9 in, 1 out]
      }
      event #13 (no event record) {
        # "Update globals for recording mode and path to read log from.\nClear when logging and let NetworkTables set path for vision to\nuse."
        n240 = event-data() -> ()  [unwired: 1 in, 1 out]
        n241 = global write "WPI_DashboardLogging Global.vi" "Logging Filename"(path "") -> ()
        n242 = case shown="\"Playback\"" {
          selector: _ -> [_ _ _]
          tunnel: w366 -> [_ w368 w376]
          tunnel: [_ _ w375] -> w363
          tunnel: [_ _ w374] -> _
          tunnel: w361 -> [_ _ w372]
          tunnel: cluster{i32, i32} {-250, 170} -> [_ _ w371]
          tunnel: [_ _ T20 {"Image Size"=TRUE, "Image Type"=TRUE, "Pixel Value"=TRUE, "ROI Information"=TRUE, "Zoom Factor"=FALSE} ("Image Information Shown:All Elements")] -> _
          tunnel: [_ _ TRUE ("Zoom Factor")] -> _
          frame Default {
          }
          frame "Stop", "Record" {
            # "Place Window too"
            n243 = invoke class="VI" method="FP.Close"(reference=w368) -> (reference out=w367:refnum<vi>)  [unwired: 2 in, 2 out]
            n244 = invoke class="VI" method="Abort VI"(reference=w367) -> ()  [unwired: 2 in, 3 out]
          }
          frame "Playback" {
            n245 = call "Open Playback Panel.vi"("Offset"=w371, "DB VI Ref"=w372, "Playback in"=w376) -> ("Playback out"=w373:refnum<vi>)  [unwired: 8 in]
            n246 = register-events(w373) -> (reference out=w375:refnum<event-registration>, error out=w374:errorcluster)  [unwired: 2 in]
          }
        }
        n247 = global read "WPI_DashboardLogging Global.vi" "Recording"() -> ()  [unwired: 1 in]
        n248 = call <vilib>:"WPI_DashboardNT Log FieldName Cache.vi"("Operation"=enum16{"Lookup/Add", "Index", "Clear"}."Clear") -> ()  [unwired: 8 in, 3 out]
      }
      event Panel Close {
        (unwired) enum32{"Stop", "Record", "Playback"}."Stop" ("Rec Mode")
        # "Playback window has been closed, abort"
        n249 = event-data() -> ()  [unwired: 1 in, 4 out]
        n250 = global read "WPI_DashboardLogging Global.vi" "Recording"() -> ()  [unwired: 1 in]
        n251 = local read item#-1() -> ()  [unwired: 1 in]
      }
      event Panel Close {
        # "Abort playback window and ourself"
        n252 = event-data() -> ()  [unwired: 1 in, 4 out]
        n253 = invoke class="VI" method="FP.Close"(reference=w381) -> (reference out=w380:refnum<vi>)  [unwired: 2 in, 2 out]
        n254 = invoke class="VI" method="Abort VI"(reference=w380) -> (error out=w379:errorcluster)  [unwired: 2 in, 2 out]
        n255 = invoke class="VI" method="Abort VI"(error in=w379) -> ()  [unwired: 2 in, 3 out]
      }
      event #16 (no event record) {
        # "Enable/Disable Compression slider.\nHW USB is hard-coded into the camera"
        n256 = event-data() -> ()  [unwired: 1 in, 1 out]
        n257 = Equal?(y=u32 2 ("milliseconds to wait")) -> (x = y?=w385:bool)  [unwired: 1 in]
        n258 = Select(t=T21."Disabled and Grayed Out" ("Disabled"), s=w385, f=T21."Enabled" ("Disabled")) -> (s? t:f=w382:T21)
        n259 = property on="Compression" class="Slide (strict)"("DisabledEnum"=w382) -> ()  [unwired: 2 in, 2 out]
      }
    }
  }
  n260 = while {
    tunnel: w33 -> [w389]
    i -> [w391]
    stop <- FALSE stop-if-true
    n261 = Wait (ms)(milliseconds to wait=u32 100) -> ()  [unwired: 1 out]
    n262 = case shown="\"Playback\"" {
      selector: _ -> [_ _ _]
      tunnel: w391 -> [_ _ w406]
      tunnel: [u32 2829099 ("Base Color") u32 11141120 ("Target Color") w395] -> w388
      frame "Stop", Default {
        # "Reset the color, extra updates don't cost much"
      }
      frame "Record" {
      }
      frame "Playback" {
        # "Playback"
        n263 = Quotient & Remainder(x=w406, y=u32 50 ("milliseconds to wait")) -> (x-y*floor(x/y)=w402:u32)  [unwired: 1 out]
        n264 = Divide(x=w402, y=u32 50 ("milliseconds to wait")) -> (x/y=w399:dbl)
        n265 = Multiply(x=6.283185307179586, y=w399) -> (x*y=w404:dbl)
        n266 = Sine(x=w404) -> (sin(x)=w403:dbl)
        n267 = Absolute Value(x=w403) -> (abs(x)=w396:dbl)
        n268 = call "Interpolate RGB Color.vi"("Proportion"=w396, "Target Color"=u32 30976, "Base Color"=u32 2829099) -> ("Result Color"=w395:u32)  [unwired: 8 in]
      }
    }
    n269 = property class="Pane"(reference=w389, "PaneColor"=w388) -> ()  [unwired: 1 in, 2 out]
  }
  n270 = TCP Create Listener(10:u16 1741 ("timeout ms (25000)")) -> (3:w1:refnum<k5>)  [unwired: 4 in, 2 out]
  n271 = while {
    tunnel: w1 -> [w408]
    stop <- FALSE stop-if-true
    n272 = TCP Wait On Listener(11:w408) -> (4:w407:refnum<k5>)  [unwired: 3 in, 4 out]
    n273 = local write "TCP"(w407) -> ()
  }
  n274 = property on="On/Off" class="Bool (strict)"("Visible"=w6) -> ()  [unwired: 2 in, 2 out]
  n275 = property on="Motor" class="Clust (strict)"("Visible"=w6) -> ()  [unwired: 2 in, 2 out]
  n276 = property on="Progress" class="Clust (strict)"("Visible"=w6) -> ()  [unwired: 2 in, 2 out]
  n277 = property on="Test Ring" class="Ring (strict)"("Visible"=w6) -> ()  [unwired: 2 in, 2 out]
  n278 = property on="Rev/Fwd" class="Clust (strict)"("Visible"=w6) -> ()  [unwired: 2 in, 2 out]
  n279 = property on="Camera Settings" class="Clust (strict)"("Visible"=w6) -> ()  [unwired: 2 in, 2 out]
  n280 = local write "DB Camera Config"(w6) -> ()
  n281 = global read "WPI_DashboardLogging Global.vi" "Recording"() -> ()  [unwired: 1 in]
  n282 = local read item#-1() -> ()  [unwired: 1 in]
